vi "Delete Wfm Header.vi"(8 "error in (no error)":errorcluster, 10 "Metadata":string, 11 "TCP Writer in":refnum<class "TCP Writer.lvclass">) -> (0 "error out":errorcluster, 3 "TCP Writer out":refnum<class "TCP Writer.lvclass">)   [LabVIEW 2012, in "TCP Classes.lvlib" / "TCP Writer.lvclass"]
uses:
  TCP Writer.lvclass
  TCP Writer.lvclass/TCP Writer.ctl
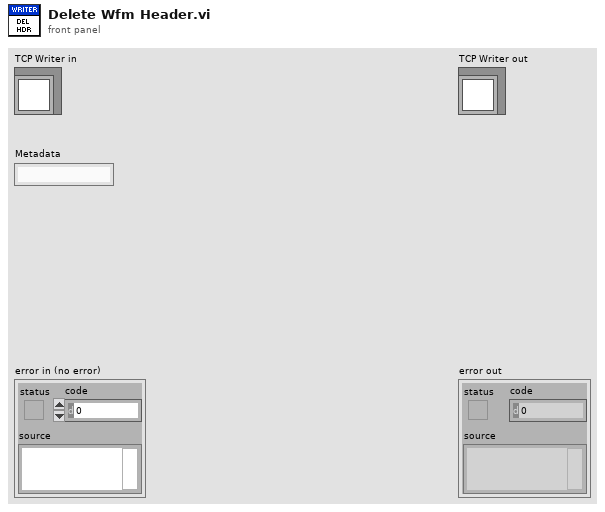
[diagram p1: front panel]
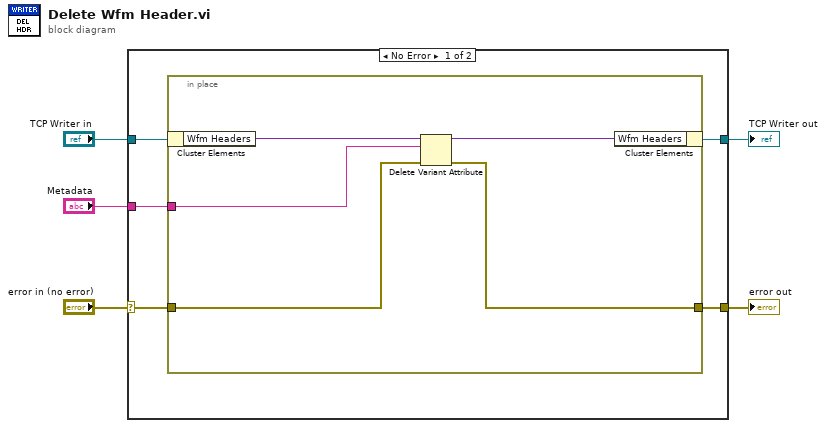
[diagram p0: block diagram]
diagram:
  n1 = case shown="No Error" "error in (no error)" {
    selector: "error in (no error)" -> [w8 w17]
    tunnel: [w6 w17] -> w4
    tunnel: [w7 w16] -> w2
    tunnel: "TCP Writer in" -> [w10 w16]
    tunnel: "Metadata" -> [w9 _]
    frame No Error {
      n2 = in-place {
        in-place-border: w9 -> [w14]
        in-place-border: w8 -> [w13]
        in-place-border: [w11] -> w6
        n3 = in-place-cluster #1(w10) -> ("Wfm Headers"=w15:variant)
        n4 = Delete Variant Attribute(4:w13, 6:w14, 7:w15) -> (0:w11:errorcluster, 3:w12:variant)  [unwired: 1 out]
        n5 = in-place-cluster #1("Wfm Headers"=w12) -> (w7:refnum<class "TCP Writer.lvclass">)
      }
    }
    frame Error {
    }
  }
  "error out" <- w4
  "TCP Writer out" <- w2
